vi "Set FFT Size.vi"(8 "error in (no error)":errorcluster, 10 "FFT Size":T1={"FFT Size"=1048576}, 11 "Application Manager in":refnum<class "Application Manager.lvclass">) -> (0 "error out":errorcluster, 3 "Application Manager out":refnum<class "Application Manager.lvclass">)   [LabVIEW 2020, in "Application Manager.lvlib" / "Application Manager.lvclass"]
uses:
  Application Manager.lvclass
  Signal Analysis/Signal Analysis/FFT Size.ctl
  Application Manager.lvclass/Application Manager.ctl
  Signal Analysis/Signal Analysis Messages/Set FFT Size Msg/Set FFT Size Msg.lvclass/Set FFT Size Msg.ctl
  <vilib>/ActorFramework/Message Enqueuer/Message Enqueuer.lvclass/Message Enqueuer.ctl
  <vilib>/ActorFramework/Message Enqueuer/Enqueue.vi
  Signal Analysis/Signal Analysis Messages/Set FFT Size Msg/Set FFT Size Msg.lvclass
  C:/Program Files/National Instruments/LabVIEW 2025/vi.lib/ActorFramework/Message/Message.lvclass
  <vilib>/ActorFramework/Message Priority Queue/Priority Enqueue.vi
  Signal Analysis/Signal Analysis/Signal Analysis.lvclass
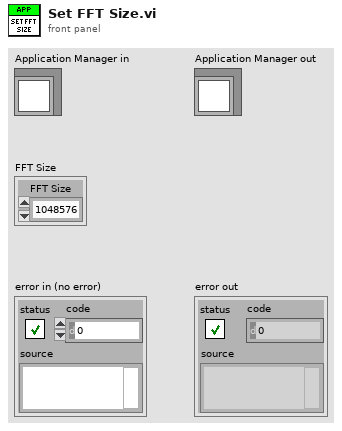
[diagram p1: front panel]
types:
  T1 = typedef "Signal Analysis.lvlib/Signal Analysis.lvclass/FFT Size.ctl" = cluster{"FFT Size":i32}
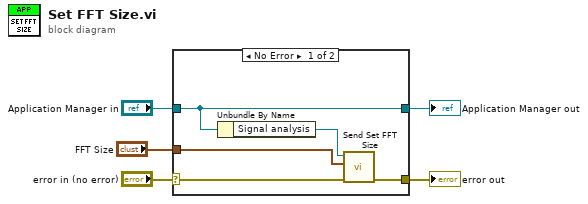
[diagram p0: block diagram]
diagram:
  n1 = case shown="No Error" "error in (no error)" {
    selector: "error in (no error)" -> [w9 w12]
    tunnel: [w6 w12] -> w4
    tunnel: [w10 w11] -> w2
    tunnel: "Application Manager in" -> [w10 w11]
    tunnel: "FFT Size" -> [w8 _]
    frame No Error {
      n2 = Unbundle By Name(w10) -> ("Signal analysis"=w7:refnum<class "Message Enqueuer.lvclass">)
      n3 = call "Send Set FFT Size.vi"("error in (no error)"=w9, "FFT Size"=w8, "Message Enqueuer"=w7) -> ("error out"=w6:errorcluster)  [unwired: 7 in, 1 out]
    }
    frame Error {
    }
  }
  "error out" <- w4
  "Application Manager out" <- w2
